vi "Live imaging window queue handler.vi"(8 "error in (no error)":errorcluster, 9 "Sim":bool, 10 "timeout in ms":i32, 11 "Queue in":T1) -> (1 "timed out?":bool, 2 "Frame rate (Hz)":dbl format="Acquisition frame rate: %.1f fps", 3 "Element to queue":T2)   [LabVIEW 2020]
uses:
  Live graphs queue/Typedefs/Live imaging queue element.ctl
  <vilib>/vision/Image Controls.llb/IMAQ Image.ctl
  Typedefs/Live graph data queue ref.ctl
  Typedefs/Read Write Enum.ctl
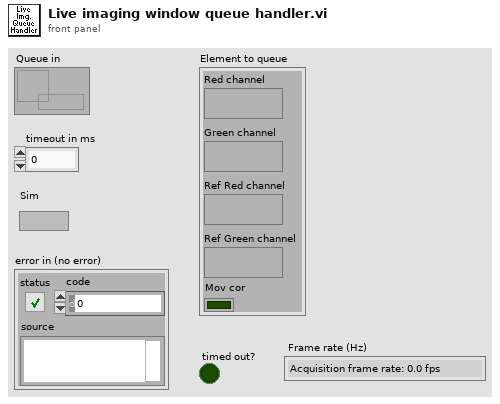
[diagram p1: front panel]
types:
  T1 = typedef "Live graph data queue ref.ctl" = refnum<queue>
  T2 = typedef "Live imaging queue element.ctl" = cluster{"Red channel":T3, "Green channel":T3, "Ref Red channel":T3, "Ref Green channel":T3, "Mov cor":bool}
  T3 = typedef "IMAQ Image.ctl" = refnum<image>
  T4 = typedef "Read Write Enum.ctl" = enum16{"Read", "Write"}
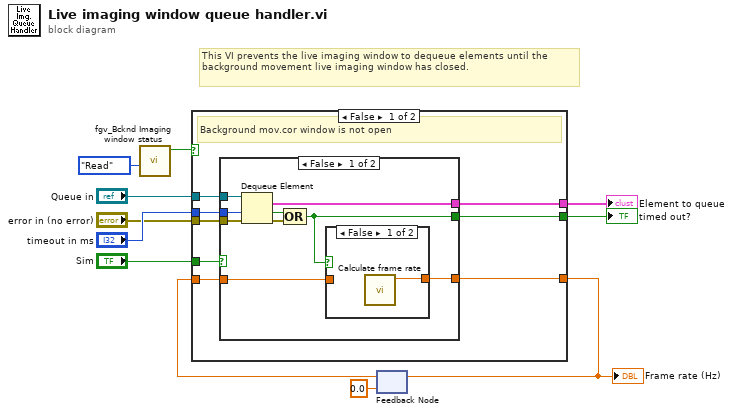
[diagram p0: block diagram]
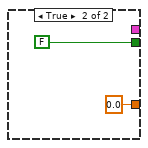
[diagram p3: hidden frame]
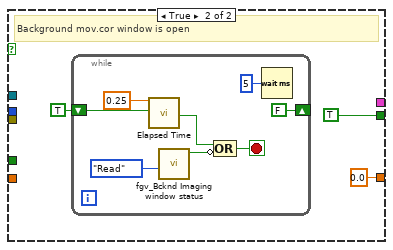
[diagram p4: hidden frame]
diagram:
  # "This VI prevents the live imaging window to dequeue elements until the background movement live imaging window has closed."
  n1 = call "fgv_Bcknd Imaging window status.vi"("Function"=Read_Write_Enum."Read") -> ("Background MovCor window is open"=w5:bool)  [unwired: 9 in, 1 out]
  n2 = feedback #1(0.0 ("Frame rate (fps)")) -> (w1:dbl)
  n3 = case shown="False" w5 {
    tunnel: "Sim" -> [w19 _]
    tunnel: "timeout in ms" -> [w18 _]
    tunnel: [w17 TRUE ("timed out?")] -> w9
    tunnel: [w16 _] -> w8
    tunnel: "error in (no error)" -> [w15 _]
    tunnel: "Queue in" -> [w14 _]
    tunnel: [w13 0.0 ("Frame rate (fps)")] -> w2
    tunnel: w1 -> [w12 _]
    frame False {
      # "Background mov.cor window is not open"
      n4 = case shown="False" w19 {
        tunnel: [w28 _] -> w16
        tunnel: w14 -> [w27 _]
        tunnel: w15 -> [w26 _]
        tunnel: w18 -> [w25 _]
        tunnel: [w22 FALSE ("timed out?")] -> w17
        tunnel: [w21 0.0 ("Frame rate (fps)")] -> w13
        tunnel: w12 -> [w20 _]
        frame False {
          n5 = Dequeue Element(queue=w27, timeout in ms (-1)=w25, error in (no error)=w26) -> (element=w28:T2, timed out?=w23:bool, error out=w24:errorcluster)  [unwired: 1 out]
          n6 = Compound Arithmetic op=OR(w23, w24) -> (w22:bool)
          n7 = case shown="False" w22 {
            tunnel: [w29 w30] -> w21
            tunnel: w20 -> [_ w30]
            frame False {
              n8 = call "Calculate frame rate.vi"() -> ("Frame rate (fps)"=w29:dbl)  [unwired: 11 in]
            }
            frame True {
            }
          }
        }
        frame True {
        }
      }
    }
    frame True {
      # "Background mov.cor window is open"
      n9 = while {
        shift-right: [FALSE] -> _
        shift-left: TRUE -> [w43]
        stop <- w36 stop-if-true
        n10 = call "Elapsed Time"("Time Target (s)"=0.25, "Reset"=w43) -> ("Time has Elapsed"=w38:bool)  [unwired: 10 in, 7 out]
        n11 = call "fgv_Bcknd Imaging window status.vi"("Function"=Read_Write_Enum."Read") -> ("Background MovCor window is open"=w37:bool)  [unwired: 9 in, 1 out]
        n12 = Compound Arithmetic op=OR(w38, invert w37) -> (w36:bool)
        n13 = Wait (ms)(milliseconds to wait=u32 5 ("millisecond timer value")) -> ()  [unwired: 1 out]
      }
    }
  }
  "timed out?" <- w9
  "Element to queue" <- w8
  "Frame rate (Hz)" <- w2
  n14 = feedback-in #1(w2) -> ()
